vi "(SubVI) Calculate xy correlation.vi"(10 "y position (delete y fit error)":dbl[](array[numeric]), 11 "x position (delete x fit error)":dbl[](array[numeric])) -> (3 "Numeric":dbl)   [LabVIEW 2016]
uses:
  <vilib>/Analysis/baseanly.llb/Mean (DBL).vi
  <vilib>/Analysis/NI_AALBase.lvlib
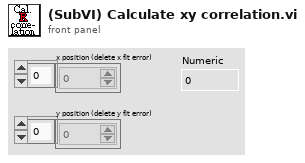
[diagram p1: front panel]
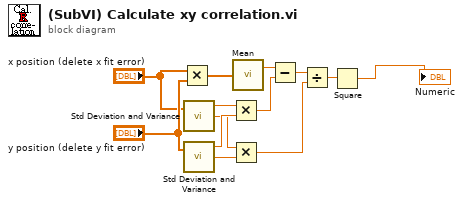
[diagram p0: block diagram]
diagram:
  n1 = Multiply(x="x position (delete x fit error)", y="y position (delete y fit error)") -> (x*y=w12:dbl[])
  n2 = call <vilib>:"Std Deviation and Variance.vi"("X"="x position (delete x fit error)") -> ("mean"=w7:dbl, "standard deviation"=w5:dbl)  [unwired: 1 in, 1 out]
  n3 = call <vilib>:"Std Deviation and Variance.vi"("X"="y position (delete y fit error)") -> ("mean"=w8:dbl, "standard deviation"=w6:dbl)  [unwired: 1 in, 1 out]
  n4 = Multiply(x=w7, y=w8) -> (x*y=w9:dbl)
  n5 = Multiply(x=w5, y=w6) -> (x*y=w4:dbl)
  n6 = call-poly <vilib>:"Mean.vi"("X"=w12) -> ("mean"=w13:dbl)  [unwired: 1 out]
  n7 = Subtract(x=w13, y=w9) -> (x-y=w3:dbl)
  n8 = Divide(x=w3, y=w4) -> (x/y=w2:dbl)
  n9 = Square(x=w2) -> (x^2=→"Numeric":dbl)
